vi "Connect Channel.vi"(7 "Configuration Entry":string, 8 "error in (no error)":errorcluster, 11 "Configuration Parameters":string[](array[string])) -> (0 "error out":errorcluster, 2 "Logic Entry":T1, 3 "Configuration Entry":T1)   [LabVIEW 2021, in "Python Orchestration.lvlib"]
uses:
  Python Orchestration.lvlib
  Typedef/Scripted Line.ctl
  CIFCore/Common/Typedef/Errors.ctl
  <vilib>/CIF Foundation/CIF Utilities/Errors/Append Error Location.vi
  CIFCore/Common/CIFCoreCommon.lvlib
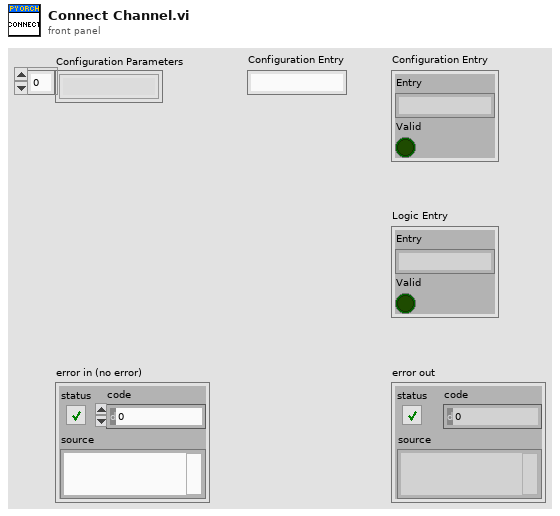
[diagram p1: front panel]
types:
  T1 = typedef "Python Orchestration.lvlib/Scripted Line.ctl" = cluster{"Entry":string, "Valid":bool}
  T2 = typedef "CIFCoreCommon.lvlib/Errors.ctl" = enum16{"Invalid Clock ID", "Long Sleep", "gRPC Server Not Found", "Config Parse", "Timestamp Wrap", "Delayed Execution", "Duplicate Channel", "Missing Channel", "Incorrect Type", "Flatten Error", "Unflatten Data", "Unique Name", "Plugin Not Found", "Plugin Type Not Found", "Plugin Version Not Found", "Manager Not Found", "Numerical Issue", "Time Jump", "Clock ID Match", "Channel Length", "Plugin Connection", "gRPC Server Connection", "PPL Name Match", "Build", "Config Log Parse", "Plugin Load", "UI Subpanel Load"}
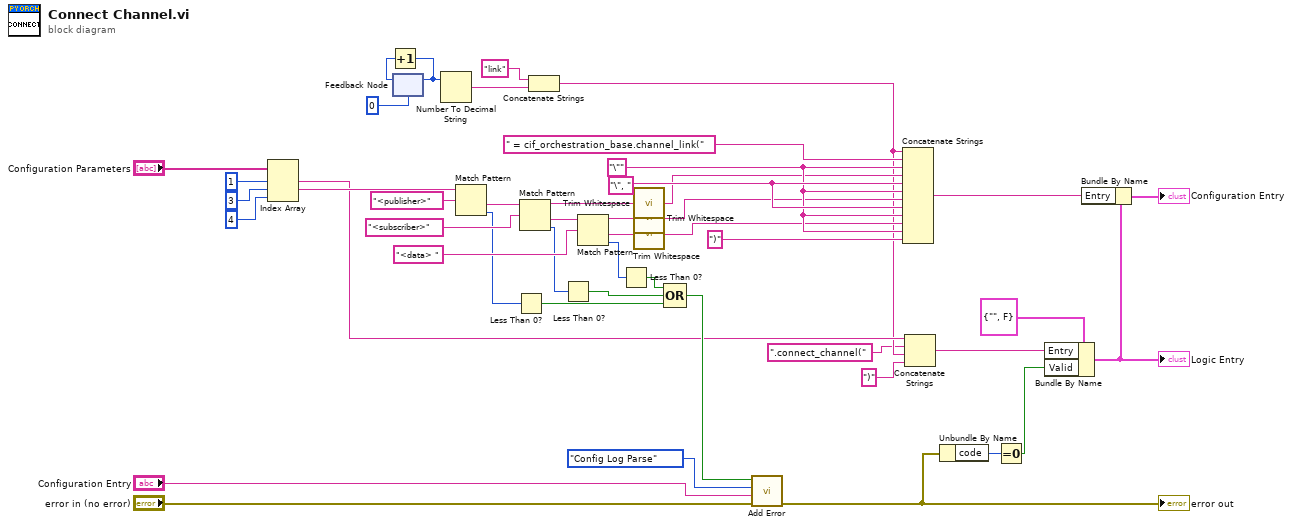
[diagram p0: block diagram]
diagram:
  w35 = "\", "
  w33 = "\""
  n1 = Index Array(array="Configuration Parameters", index #1=1 ("index"), index #2=3 ("index"), index #3=4 ("index")) -> (element #1=w7:string, element #2=w26:string)  [unwired: 1 out]
  n2 = feedback #1(u16 0) -> (w30:u16)
  n3 = Increment(x=w30) -> (x+1=w29:u16)
  n4 = feedback-in #1(w29) -> ()
  n5 = Number To Decimal String(number=w29) -> (decimal integer string=w27:string)  [unwired: 1 in]
  n6 = Match Pattern(string=w26, regular expression="<publisher>") -> (after substring=w36:string, offset past match=w11:i32)  [unwired: 1 in, 2 out]
  n7 = Less Than 0?(x=w11) -> (x < 0?=w10:bool)
  n8 = Match Pattern(string=w36, regular expression="<subscriber>") -> (before substring=w24:string, after substring=w22:string, offset past match=w12:i32)  [unwired: 1 in, 1 out]
  n9 = Concatenate Strings("link" ("string"), w27) -> (w6:string)
  n10 = Less Than 0?(x=w12) -> (x < 0?=w9:bool)
  n11 = Match Pattern(string=w22, regular expression="<data> ") -> (before substring=w20:string, after substring=w18:string, offset past match=w13:i32)  [unwired: 1 in, 1 out]
  n12 = Less Than 0?(x=w13) -> (x < 0?=w8:bool)
  n13 = call <vilib>:"Trim Whitespace.vi"("string"=w24) -> ("trimmed string"=w23:string)  [unwired: 1 in]
  n14 = call <vilib>:"Trim Whitespace.vi"("string"=w20) -> ("trimmed string"=w19:string)  [unwired: 1 in]
  n15 = call <vilib>:"Trim Whitespace.vi"("string"=w18) -> ("trimmed string"=w17:string)  [unwired: 1 in]
  n16 = Compound Arithmetic op=OR(w8, w9, w10) -> (w47:bool)
  n17 = call "Add Error.vi"("error in (no error)"="error in (no error)", "String to Append"="Configuration Entry", "Error"=Errors."Config Log Parse", "Insert Error"=w47) -> ("error out"=w43:errorcluster)  [unwired: 7 in]
  "error out" <- w43
  n18 = Concatenate Strings(w6, " = cif_orchestration_base.channel_link(", w33, w23, w35, w33, w19, w35, w33, w17, w33, ")" ("string")) -> (w15:string)
  n19 = Concatenate Strings(w7, ".connect_channel(" ("string"), w6, ")" ("string")) -> (w14:string)
  n20 = Unbundle By Name(w43) -> ("code"=w42:i32)
  n21 = Equal To 0?(x=w42) -> (x = 0?=w41:bool)
  n22 = Bundle By Name(cluster=T1 {"Entry"="", "Valid"=FALSE} ("Logic Entry"), "Entry"=w14, "Valid"=w41) -> (w1:T1)
  "Logic Entry" <- w1
  n23 = Bundle By Name(cluster=w1, "Entry"=w15) -> (→"Configuration Entry":T1)
